vi "BoolSelection.vi"() -> (0 "BoolSelection":bool[][](array[boolean]))   [LabVIEW 2022 SP3]
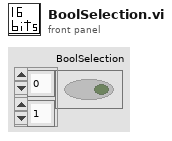
[diagram p1: front panel]
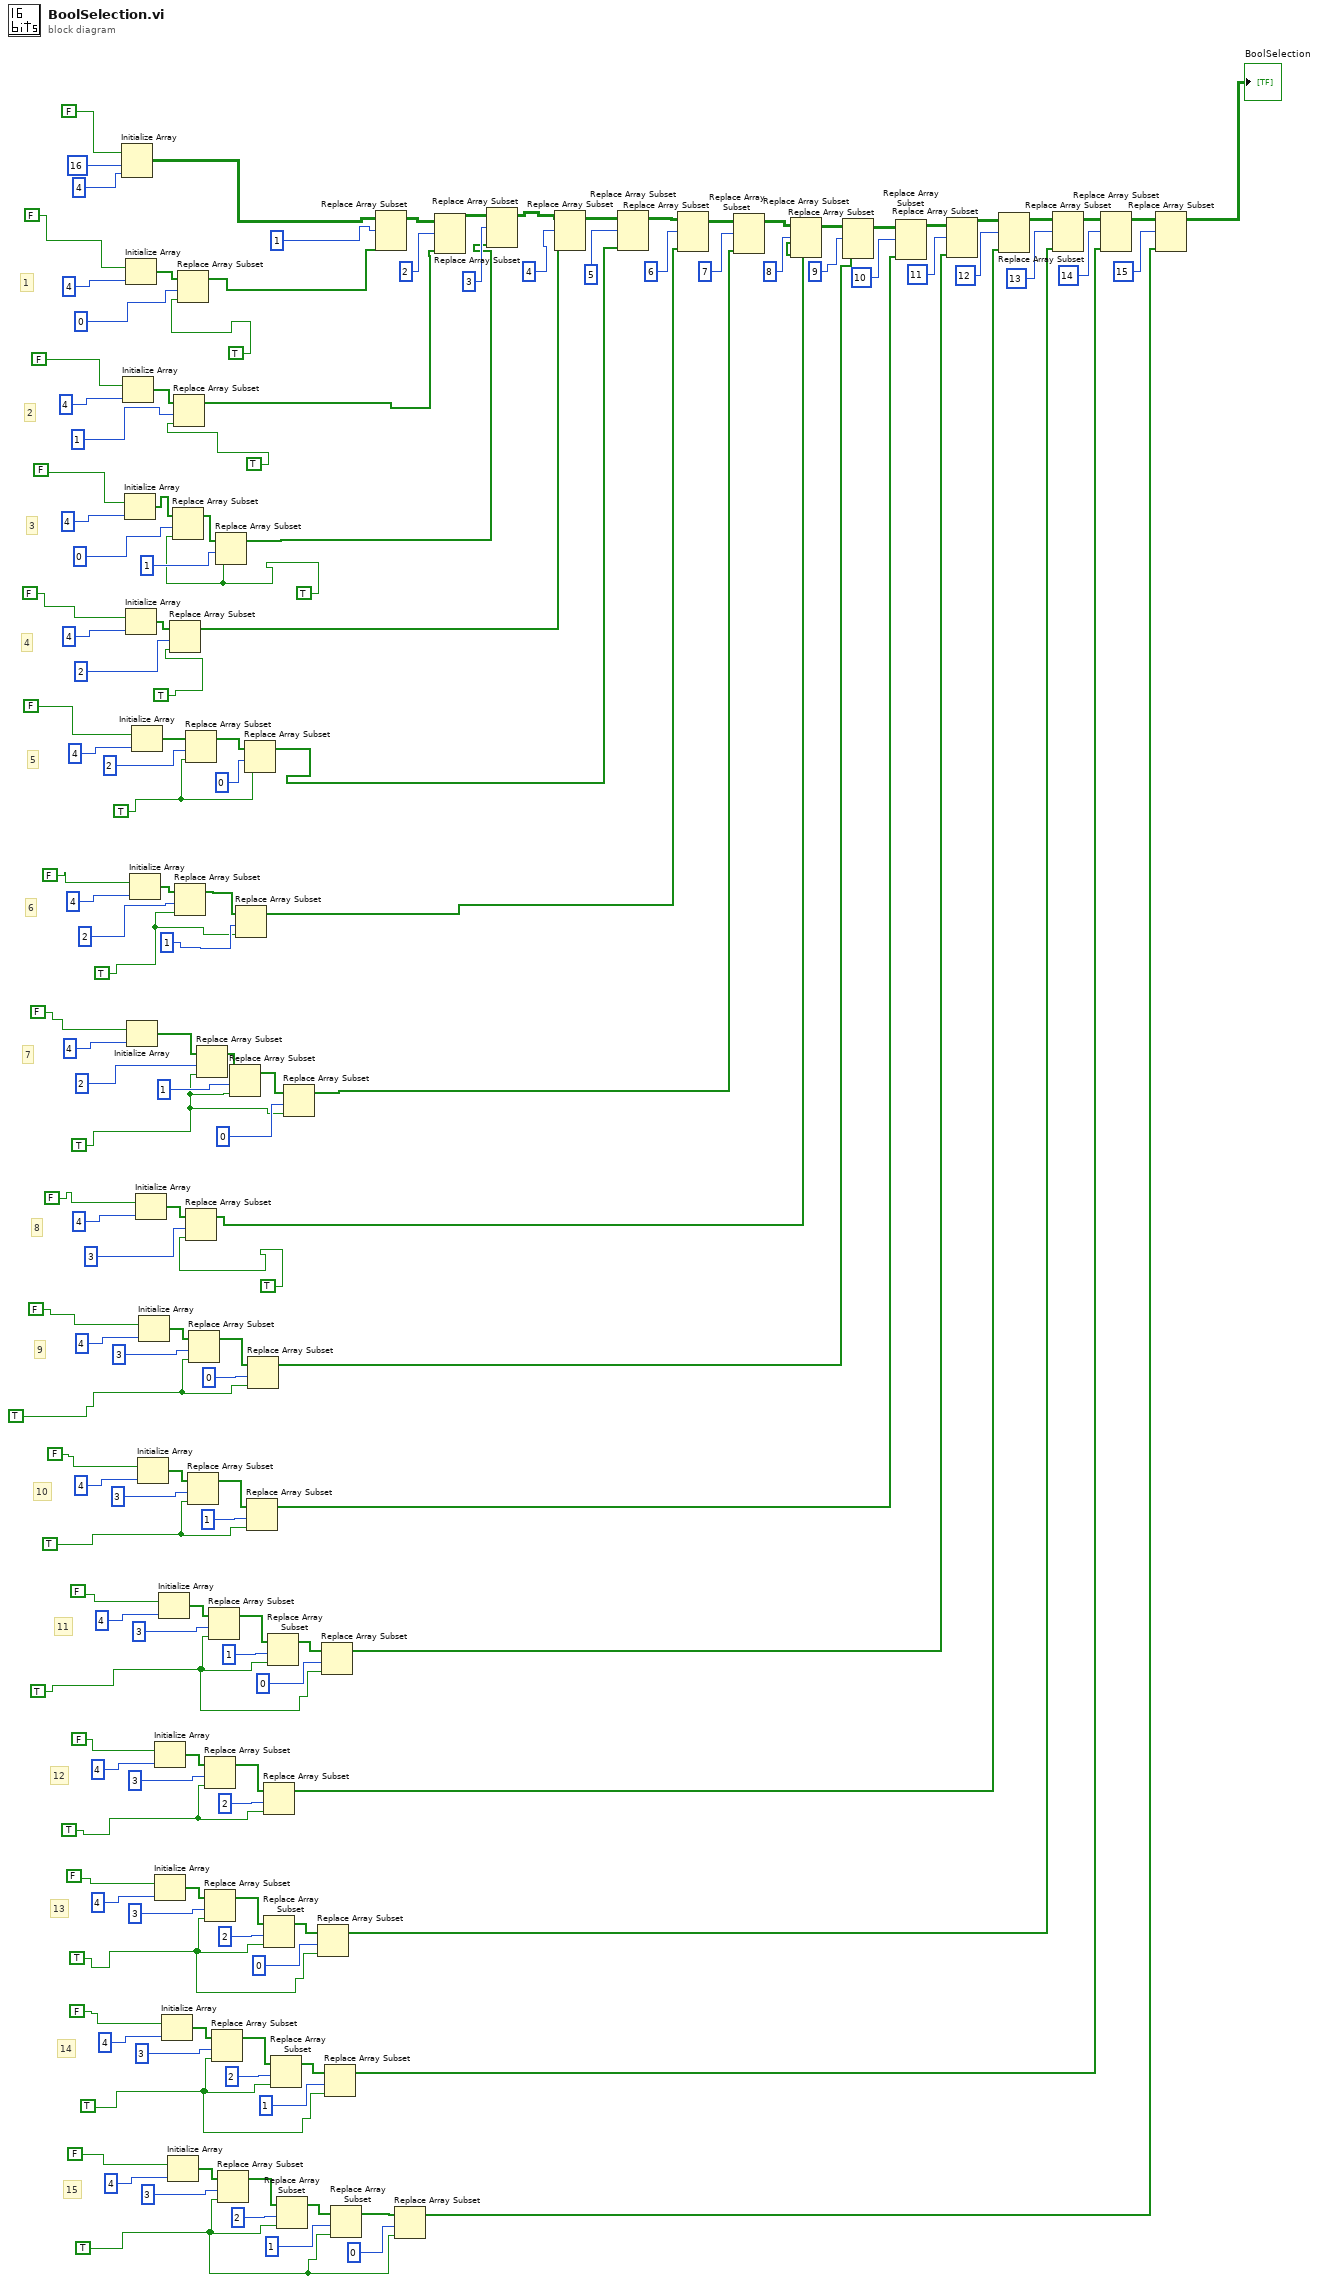
[diagram p0: block diagram]
diagram:
  w4 = TRUE
  w6 = TRUE
  w7 = TRUE
  w8 = TRUE
  w10 = TRUE
  w11 = TRUE
  w12 = TRUE
  w13 = TRUE
  w14 = TRUE
  w15 = TRUE
  w16 = TRUE
  # "15"
  # "14"
  # "13"
  # "12"
  # "11"
  # "10"
  # "9"
  # "8"
  # "7"
  # "6"
  # "5"
  # "4"
  # "3"
  # "2"
  # "1"
  n1 = Initialize Array(FALSE, 16, 4) -> (w148:bool[][])
  n2 = Initialize Array(FALSE, 4) -> (w128:bool[])
  n3 = Initialize Array(FALSE, 4) -> (w125:bool[])
  n4 = Initialize Array(FALSE, 4) -> (w131:bool[])
  n5 = Initialize Array(FALSE, 4) -> (w120:bool[])
  n6 = Initialize Array(FALSE, 4) -> (w108:bool[])
  n7 = Initialize Array(FALSE, 4) -> (w113:bool[])
  n8 = Initialize Array(FALSE, 4) -> (w118:bool[])
  n9 = Initialize Array(FALSE, 4) -> (w101:bool[])
  n10 = Initialize Array(FALSE, 4) -> (w92:bool[])
  n11 = Initialize Array(FALSE, 4) -> (w97:bool[])
  n12 = Initialize Array(FALSE, 4) -> (w80:bool[])
  n13 = Initialize Array(FALSE, 4) -> (w63:bool[])
  n14 = Initialize Array(FALSE, 4) -> (w87:bool[])
  n15 = Initialize Array(FALSE, 4) -> (w56:bool[])
  n16 = Initialize Array(FALSE, 4) -> (w49:bool[])
  n17 = Replace Array Subset(array=w120, new element=TRUE, index=2) -> (w121:bool[])
  n18 = Replace Array Subset(array=w125, new element=w4, index=0) -> (w124:bool[])
  n19 = Replace Array Subset(array=w128, new element=TRUE, index=1) -> (w129:bool[])
  n20 = Replace Array Subset(array=w113, new element=w7, index=2) -> (w110:bool[])
  n21 = Replace Array Subset(array=w131, new element=TRUE, index=0) -> (w132:bool[])
  n22 = Replace Array Subset(array=w118, new element=w6, index=2) -> (w116:bool[])
  n23 = Replace Array Subset(array=w101, new element=TRUE, index=3) -> (w100:bool[])
  n24 = Replace Array Subset(array=w92, new element=w11, index=3) -> (w90:bool[])
  n25 = Replace Array Subset(array=w97, new element=w10, index=3) -> (w95:bool[])
  n26 = Replace Array Subset(array=w108, new element=w8, index=2) -> (w106:bool[])
  n27 = Replace Array Subset(array=w80, new element=w13, index=3) -> (w78:bool[])
  n28 = Replace Array Subset(array=w63, new element=w14, index=3) -> (w61:bool[])
  n29 = Replace Array Subset(array=w87, new element=w12, index=3) -> (w85:bool[])
  n30 = Replace Array Subset(array=w56, new element=w15, index=3) -> (w54:bool[])
  n31 = Replace Array Subset(array=w124, new element=w4, index=1) -> (w123:bool[])
  n32 = Replace Array Subset(array=w49, new element=w16, index=3) -> (w47:bool[])
  n33 = Replace Array Subset(array=w106, new element=w8, index=1) -> (w103:bool[])
  n34 = Replace Array Subset(array=w110, new element=w7, index=1) -> (w111:bool[])
  n35 = Replace Array Subset(array=w116, new element=w6, index=0) -> (w115:bool[])
  n36 = Replace Array Subset(array=w90, new element=w11, index=1) -> (w67:bool[])
  n37 = Replace Array Subset(array=w95, new element=w10, index=0) -> (w68:bool[])
  n38 = Replace Array Subset(array=w78, new element=w13, index=2) -> (w65:bool[])
  n39 = Replace Array Subset(array=w61, new element=w14, index=2) -> (w58:bool[])
  n40 = Replace Array Subset(array=w85, new element=w12, index=1) -> (w82:bool[])
  n41 = Replace Array Subset(array=w54, new element=w15, index=2) -> (w51:bool[])
  n42 = Replace Array Subset(array=w47, new element=w16, index=2) -> (w44:bool[])
  n43 = Replace Array Subset(array=w103, new element=w8, index=0) -> (w104:bool[])
  n44 = Replace Array Subset(array=w58, new element=w14, index=0) -> (w35:bool[])
  n45 = Replace Array Subset(array=w82, new element=w12, index=0) -> (w66:bool[])
  n46 = Replace Array Subset(array=w51, new element=w15, index=1) -> (w34:bool[])
  n47 = Replace Array Subset(array=w44, new element=w16, index=1) -> (w43:bool[])
  n48 = Replace Array Subset(array=w148, new element=w132, index (row)=1) -> (w146:bool[][])  [unwired: 1 in]
  n49 = Replace Array Subset(array=w43, new element=w16, index=0) -> (w33:bool[])
  n50 = Replace Array Subset(array=w146, new element=w129, index (row)=2) -> (w143:bool[][])  [unwired: 1 in]
  n51 = Replace Array Subset(array=w143, new element=w123, index (row)=3) -> (w141:bool[][])  [unwired: 1 in]
  n52 = Replace Array Subset(array=w141, new element=w121, index (row)=4) -> (w139:bool[][])  [unwired: 1 in]
  n53 = Replace Array Subset(array=w139, new element=w115, index (row)=5) -> (w137:bool[][])  [unwired: 1 in]
  n54 = Replace Array Subset(array=w137, new element=w111, index (row)=6) -> (w135:bool[][])  [unwired: 1 in]
  n55 = Replace Array Subset(array=w135, new element=w104, index (row)=7) -> (w133:bool[][])  [unwired: 1 in]
  n56 = Replace Array Subset(array=w133, new element=w100, index (row)=8) -> (w76:bool[][])  [unwired: 1 in]
  n57 = Replace Array Subset(array=w76, new element=w68, index (row)=9) -> (w74:bool[][])  [unwired: 1 in]
  n58 = Replace Array Subset(array=w74, new element=w67, index (row)=10) -> (w73:bool[][])  [unwired: 1 in]
  n59 = Replace Array Subset(array=w73, new element=w66, index (row)=11) -> (w72:bool[][])  [unwired: 1 in]
  n60 = Replace Array Subset(array=w72, new element=w65, index (row)=12) -> (w41:bool[][])  [unwired: 1 in]
  n61 = Replace Array Subset(array=w41, new element=w35, index (row)=13) -> (w40:bool[][])  [unwired: 1 in]
  n62 = Replace Array Subset(array=w40, new element=w34, index (row)=14) -> (w39:bool[][])  [unwired: 1 in]
  n63 = Replace Array Subset(array=w39, new element=w33, index (row)=15) -> (→"BoolSelection":bool[][])  [unwired: 1 in]
